vi "test2.vi"() -> ()   [LabVIEW 2020]
panel:
  in  "Stop":bool
  in  "Temperatures":T1
  out "Process Temperature \nChart":dbl(graph)
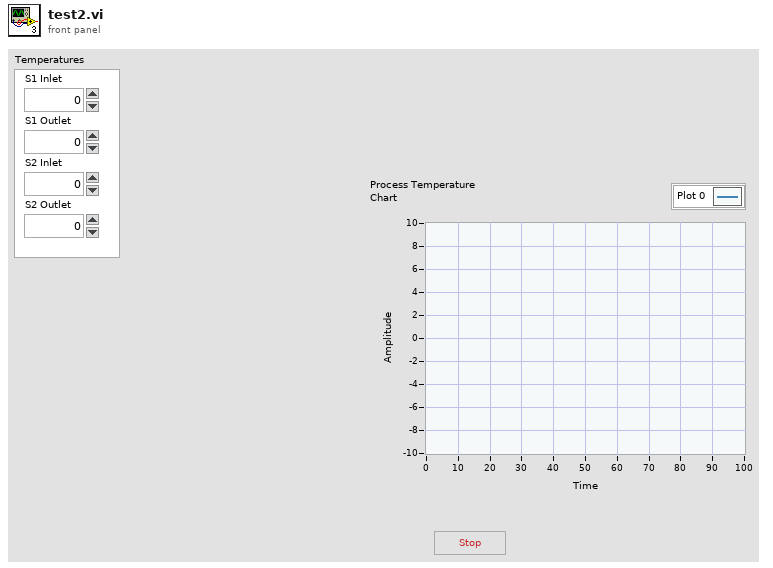
[diagram p1: front panel]
types:
  T1 = cluster{"S1 Inlet":dbl, "S1 Outlet":dbl, "S2 Inlet":dbl, "S2 Outlet":dbl}
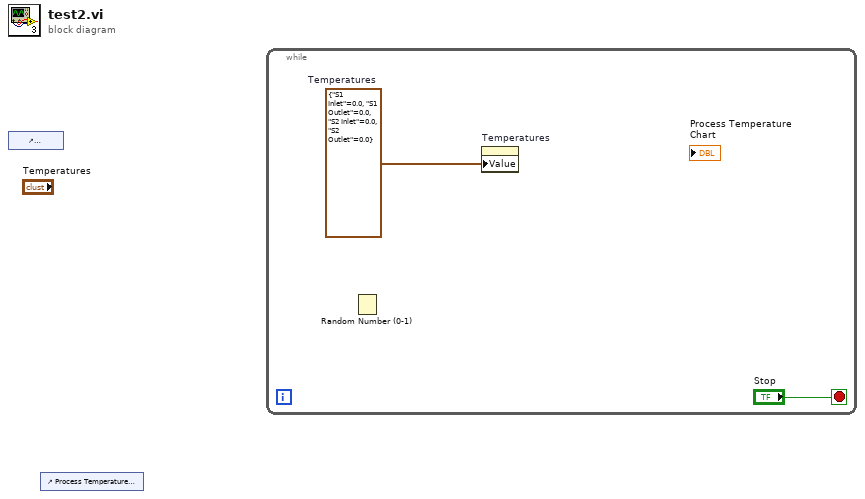
[diagram p0: block diagram]
diagram:
  n1 = control-ref of="Temperatures"() -> ()  [unwired: 1 out]
  n2 = control-ref of="Process Temperature \nChart"() -> ()  [unwired: 1 out]
  n3 = while {
    stop <- "Stop" stop-if-true
    w1 = T1 {"S1 Inlet"=0.0, "S1 Outlet"=0.0, "S2 Inlet"=0.0, "S2 Outlet"=0.0}  # Temperatures
    n4 = Random Number (0-1)() -> ()  [unwired: 1 out]
    n5 = property on="Temperatures" class="Clust (strict)"("Value"=w1) -> ()  [unwired: 2 in, 2 out]
  }
